vi "Program.vi"() -> ()   [LabVIEW 2023]
uses:
  <vilib>/measure/NI_MAPro.lvlib
  Controls/Enum 2 - States.ctl
  <vilib>/sound2/lvsound2.llb/Sampling Mode.ctl
  <vilib>/sound2/lvsound2.llb/Sound Input Task ID.ctl
  <vilib>/sound2/lvsound2.llb/Sound File Refnum.ctl
  Controls/Enum 1.ctl
  <vilib>/sound2/lvsound2.llb/Sound Data Format.ctl
  Controls/Enum 3 - States.ctl
  Controls/UI Message.ctl
  <vilib>/sound2/lvsound2.llb/Sound Input Read (DBL).vi
  <vilib>/measure/maspectr.llb/FFT Spectrum (Mag-Phase) for N Chan.vi
  <vilib>/sound2/lvsound2.llb/Sound File Write Open.vi
  <vilib>/sound2/lvsound2.llb/Sound File Write (DBL).vi
  Controls/Parameters In.ctl
panel:
  in  "Stop":bool
  in  "Sound format":T1={"sample rate (S/s)"=48000.0, "number of channels"=2, "bits per sample"=24}
  in  "number of samples/ch":i32=12000
  in  "Play":bool
  in  "Path":path
  in  "Tab Control":enum32{"Waveform Analyzer", "Spectrum Analyzer"}(tab)
  out "Waveform Graph":waveform(dbl)[](graph)
  out "Spectrum Graph":cluster{"f0":dbl, "df":dbl, "magnitude":dbl[]}[](graph)
  in  "Zoom 2":i32(slide) scale=100.0..1.0
  in  "Zoom":i32(slide) scale=1000.0..1.0
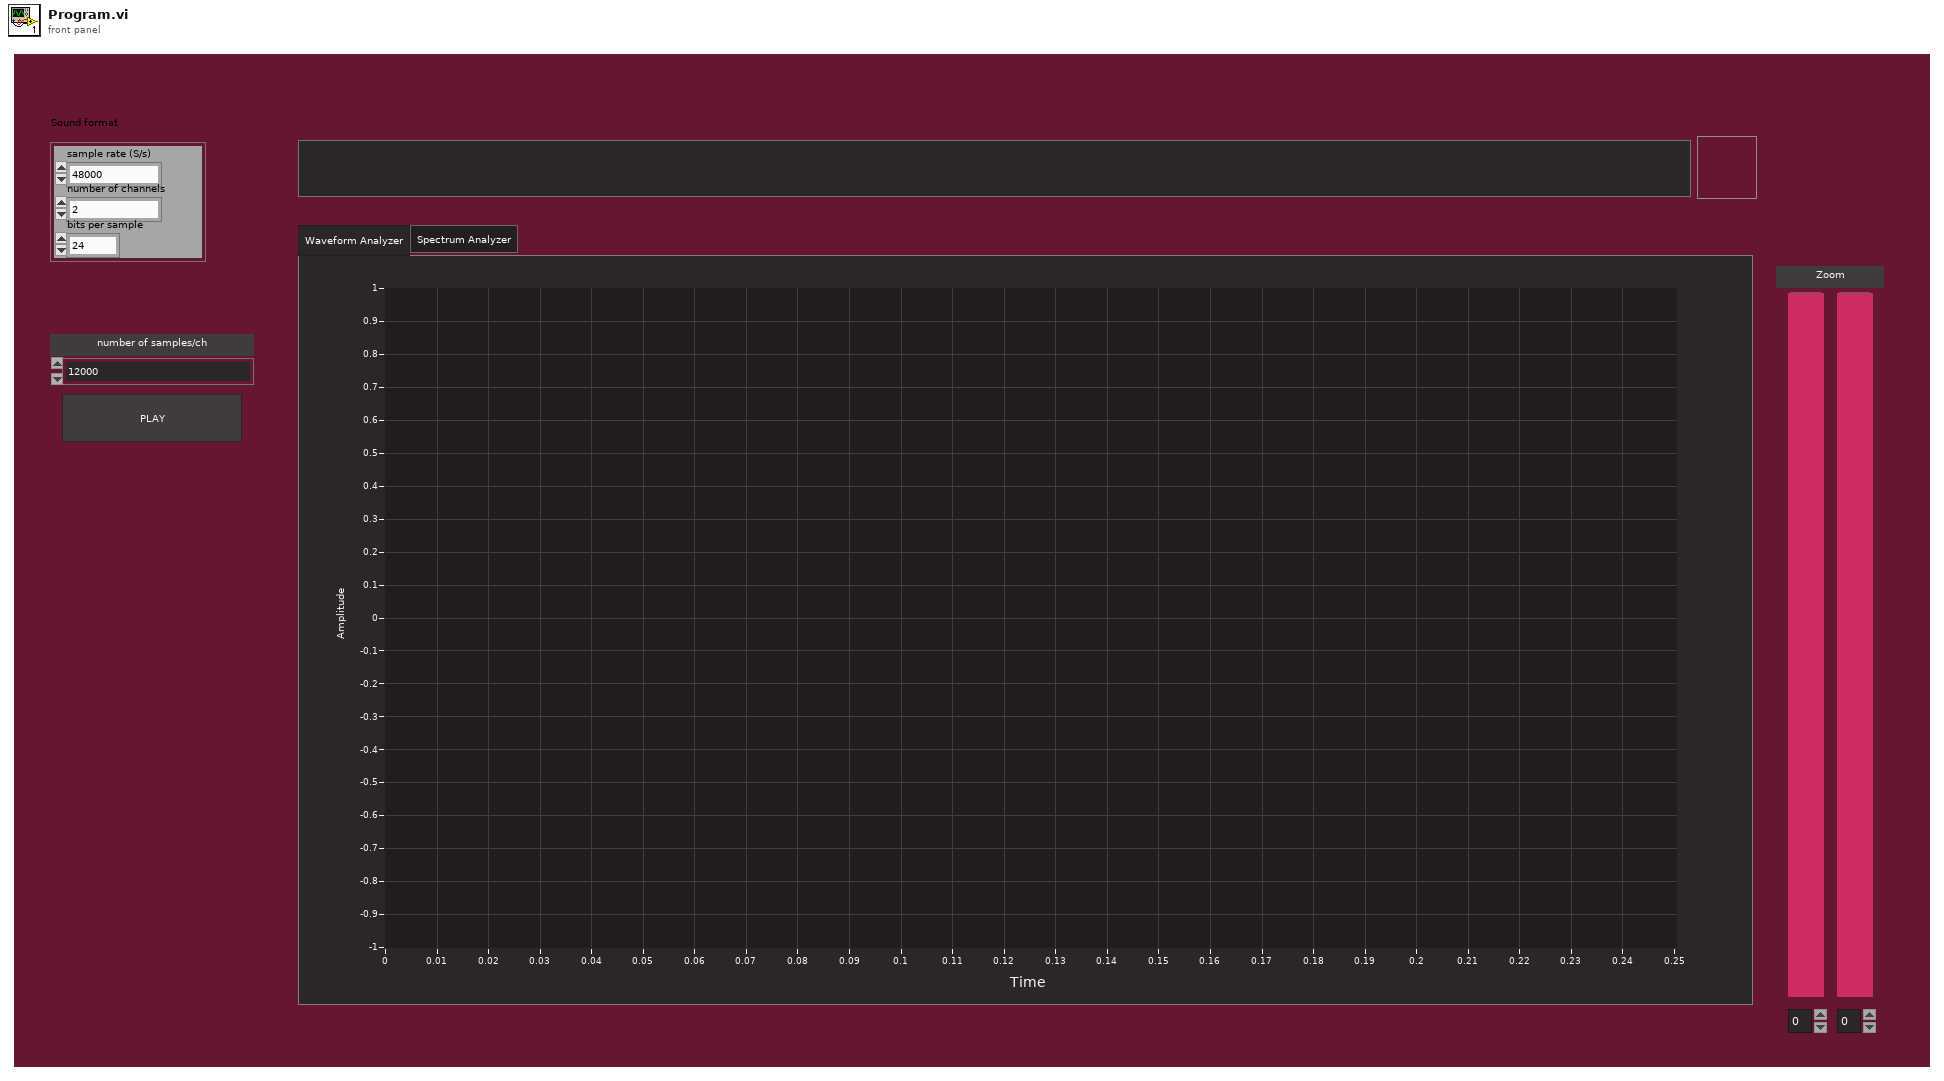
[diagram p1: front panel]
types:
  T1 = typedef "Sound Data Format.ctl" = cluster{"sample rate (S/s)":dbl, "number of channels":i32, "bits per sample":i32}
  T2 = typedef "UI Message.ctl" = cluster{"Time Signal ":waveform(dbl)[], "FFT":cluster{"f0":dbl, "df":dbl, "magnitude":dbl[]}[]}
  T3 = typedef "Enum 3 - States.ctl" = enum16{"Idle", "Init", "Analysis", "End"}
  T4 = typedef "Enum 2 - States.ctl" = enum16{"Idle", "Init", "ACQ", "End"}
  T5 = typedef "Parameters In.ctl" = cluster{"Stop":bool, "Play":bool, "number of samples/ch":i32, "sound format":T1, "Path":path}
  T6 = typedef "Enum 1.ctl" = enum16{"Set", "Get"}
  T7 = typedef "Sound File Refnum.ctl" = refnum<file>
  T8 = typedef "Sound Input Task ID.ctl" = u32
  T9 = typedef "Sampling Mode.ctl" = i32
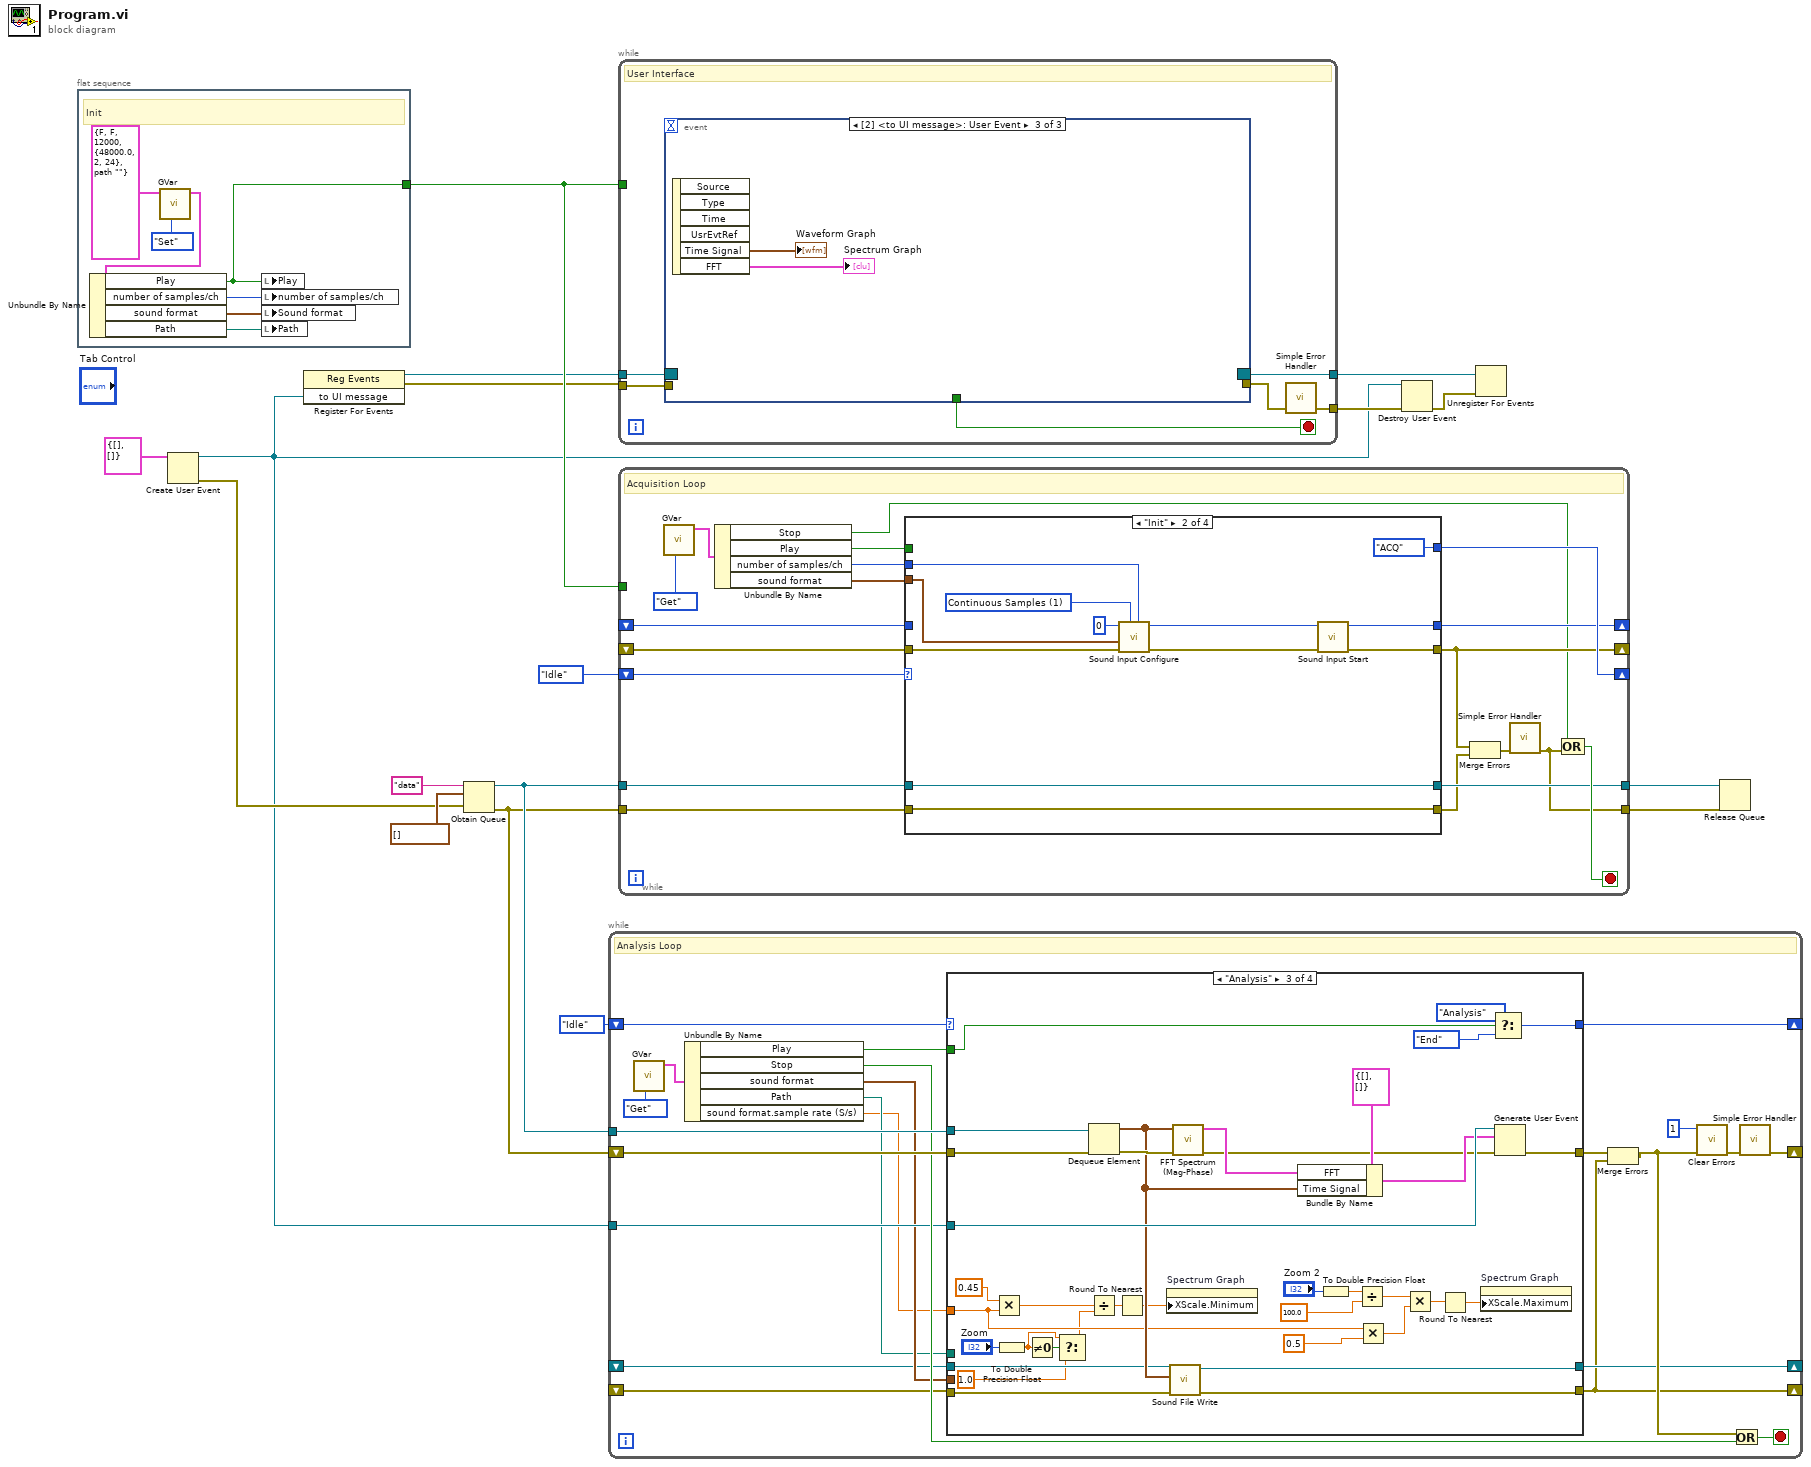
[diagram p0: block diagram]
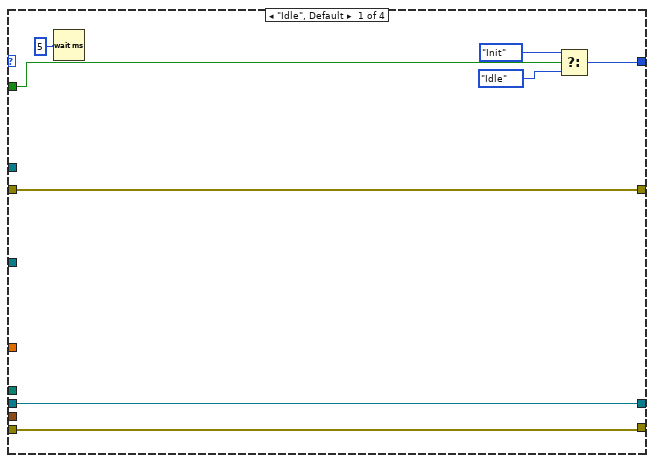
[diagram p2: hidden frame]
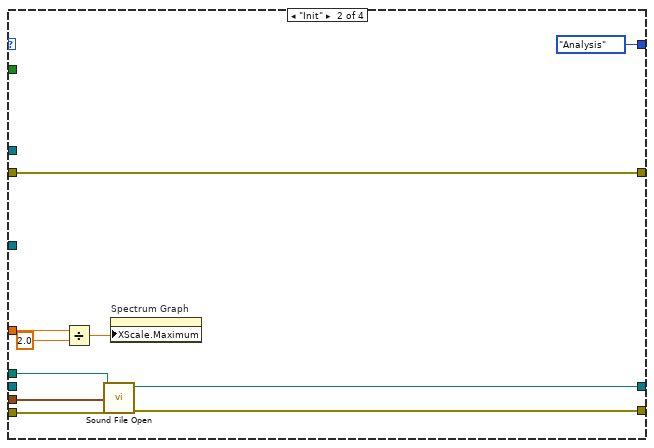
[diagram p3: hidden frame]
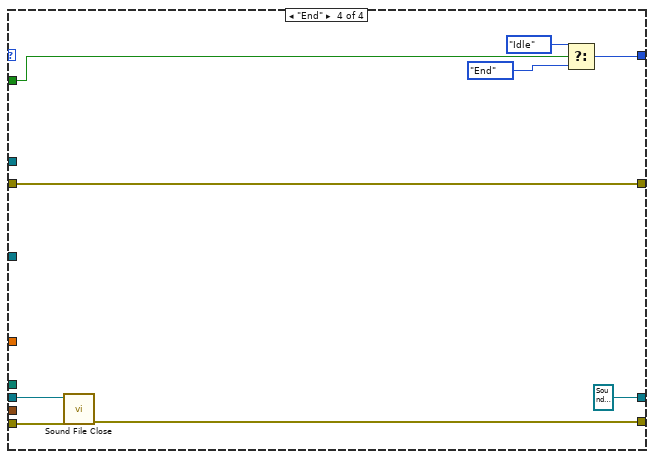
[diagram p4: hidden frame]
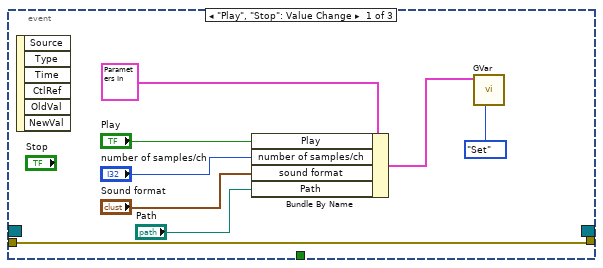
[diagram p5: hidden frame]
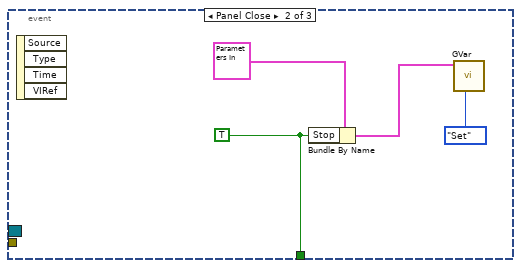
[diagram p6: hidden frame]
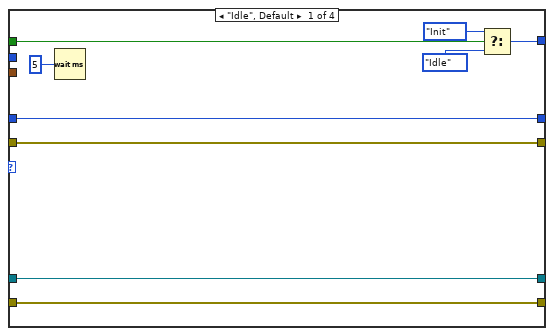
[diagram p7: hidden frame]
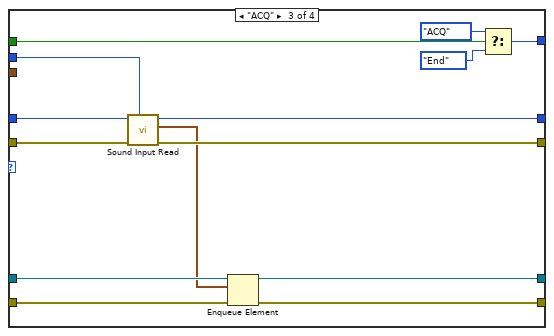
[diagram p8: hidden frame]
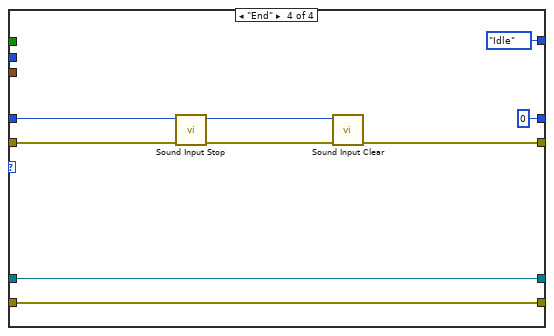
[diagram p9: hidden frame]
diagram:
  n1 = flat-sequence {
    tunnel: [w20] -> w16
    frame #0 {
      # "Init"
      n2 = call "GVar.vi"("Action"=Enum_1."Set", "Parameters In"=T5 {"Stop"=FALSE, "Play"=FALSE, "number of samples/ch"=12000, "sound format"={"sample rate (S/s)"=48000.0, "number of channels"=2, "bits per sample"=24}, "Path"=path ""}) -> ("Parameters In 2"=w23:T5)  [unwired: 9 in]
      n3 = Unbundle By Name(w23) -> ("Play"=w20:bool, "number of samples/ch"=w21:i32, "sound format"=w22:T1, "Path"=w19:path)
      n4 = local write "Play"(w20) -> ()
      n5 = local write "number of samples/ch"(w21) -> ()
      n6 = local write "Sound format"(w22) -> ()
      n7 = local write "Path"(w19) -> ()
    }
  }
  n8 = Create User Event(user event datatype=T2 {"Time Signal "=[], "FFT"=[]} ("to UI message")) -> (user event=w4:refnum<user-event>, error out=w11:errorcluster)  [unwired: 1 in]
  n9 = register-events(w4) -> (reference out=w10:refnum<event-registration>, error out=w7:errorcluster)  [unwired: 2 in]
  n10 = Obtain Queue(name (unnamed)="data", element data type=waveform(dbl)[] [] ("data"), error in (no error)=w11) -> (queue out=w13:refnum<queue>, error out=w1:errorcluster)  [unwired: 2 in, 1 out]
  n11 = while {
    tunnel: w13 -> [w45]
    shift-right: [w36] -> _
    shift-left: w1 -> [w44]
    shift-right: [w39] -> _
    shift-left: Enum_3_-_States."Idle" -> [w46]
    tunnel: w4 -> [w37]
    shift-right: [w31] -> _
    shift-left: _ -> [w27]
    shift-right: [w29] -> _
    shift-left: _ -> [w28]
    stop <- w41 stop-if-true
    # "Analysis Loop"
    n12 = call "GVar.vi"("Action"=Enum_1."Get") -> ("Parameters In 2"=w42:T5)  [unwired: 10 in]
    n13 = Unbundle By Name(w42) -> ("Play"=w38:bool, "Stop"=w40:bool, "sound format"=w33:T1, "Path"=w26:path, "sound format.sample rate (S/s)"=w25:dbl)
    n14 = case shown="\"Analysis\"" w46 {
      tunnel: w44 -> [w53 w62 w100 w101]
      tunnel: w45 -> [_ _ w99 _]
      tunnel: [w53 w62 w88 w101] -> w30
      tunnel: [w50 Enum_3_-_States."Analysis" w95 w107] -> w39
      tunnel: w38 -> [w49 _ w94 w106]
      tunnel: w37 -> [_ _ w93 _]
      tunnel: w33 -> [_ w64 _ _]
      tunnel: [w47 w63 w84 T7 refnum ("sound file refnum out")] -> w31
      tunnel: [w48 w61 w86 w103] -> w29
      tunnel: w28 -> [w48 w59 w83 w104]
      tunnel: w27 -> [w47 _ w85 w105]
      tunnel: w26 -> [_ w58 _ _]
      tunnel: w25 -> [_ w57 w70 _]
      frame "Idle", Default {
        n15 = Wait (ms)(milliseconds to wait=u32 5) -> ()  [unwired: 1 out]
        n16 = Select(t=Enum_3_-_States."Init", s=w49, f=Enum_3_-_States."Idle") -> (s? t:f=w50:T3)
      }
      frame "Init" {
        n17 = Divide(x=w57, y=2.0) -> (x/y=w55:dbl)
        n18 = call-poly <vilib>:"Sound File Open.vi"("error in (no error)"=w59, "sound format"=w64, "path"=w58) -> ("error out"=w61:errorcluster, "sound file refnum"=w63:T7)  [unwired: 7 in]
        n19 = property on="Spectrum Graph" class="WFGraph (strict)"("XScale.Maximum"=w55) -> ()  [unwired: 2 in, 2 out]
      }
      frame "Analysis" {
        n20 = Multiply(x=0.45, y=w70) -> (x*y=w81:dbl)
        n21 = To Double Precision Float(number="Zoom") -> (double precision float=w67:dbl)
        n22 = Not Equal To 0?(x=w67) -> (x != 0?=w68:bool)
        n23 = Select(t=w67, s=w68, f=1.0) -> (s? t:f=w65:dbl)
        n24 = Dequeue Element(queue=w99, error in (no error)=w100) -> (element=w87:waveform(dbl)[], error out=w98:errorcluster)  [unwired: 1 in, 2 out]
        n25 = Divide(x=w81, y=w65) -> (x/y=w73:dbl)
        n26 = Round To Nearest(number=w73) -> (nearest integer value=w72:dbl)
        n27 = property on="Spectrum Graph" class="WFGraph (strict)"("XScale.Minimum"=w72) -> ()  [unwired: 2 in, 2 out]
        n28 = call-poly <vilib>:"Sound File Write.vi"("error in (no error)"=w83, "data"=w87, "sound file refnum"=w85) -> ("error out"=w86:errorcluster, "sound file refnum out"=w84:T7)  [unwired: 7 in]
        n29 = call-poly <vilib>:"FFT Spectrum (Mag-Phase).vi"("error in (no error)"=w98, "time signals"=w87) -> ("error out"=w89:errorcluster, "magnitudes"=w92:cluster{"f0":dbl, "df":dbl, "magnitude":dbl[]}[])  [unwired: 5 in, 3 out]
        n30 = Bundle By Name(cluster=T2 {"Time Signal "=[], "FFT"=[]} ("to UI message"), "FFT"=w92, "Time Signal"=w87) -> (w90:T2)
        n31 = To Double Precision Float(number="Zoom 2") -> (double precision float=w77:dbl)
        n32 = Divide(x=w77, y=100.0) -> (x/y=w80:dbl)
        n33 = Multiply(x=w70, y=0.5) -> (x*y=w69:dbl)
        n34 = Multiply(x=w80, y=w69) -> (x*y=w75:dbl)
        n35 = Round To Nearest(number=w75) -> (nearest integer value=w74:dbl)
        n36 = property on="Spectrum Graph" class="WFGraph (strict)"("XScale.Maximum"=w74) -> ()  [unwired: 2 in, 2 out]
        n37 = Select(t=Enum_3_-_States."Analysis", s=w94, f=Enum_3_-_States."End") -> (s? t:f=w95:T3)
        n38 = Generate User Event(user event=w93, event data cluster=w90, error in=w89) -> (error out=w88:errorcluster)  [unwired: 1 in, 1 out]
      }
      frame "End" {
        n39 = call <vilib>:"Sound File Close.vi"("error in (no error)"=w104, "sound file refnum"=w105) -> ("error out"=w103:errorcluster)  [unwired: 9 in]
        n40 = Select(t=Enum_3_-_States."Idle", s=w106, f=Enum_3_-_States."End") -> (s? t:f=w107:T3)
      }
    }
    n41 = Merge Errors(w30, w29) -> (w32:errorcluster)
    n42 = call <vilib>:"Clear Errors.vi"("error in (no error)"=w32, "specific error code to clear (0: all)"=1) -> ("error out"=w34:errorcluster)  [unwired: 4 in, 1 out]
    n43 = Or(x=w32, y=w40) -> (x .or. y?=w41:bool)
    n44 = call <vilib>:"Simple Error Handler.vi"("error in (no error)"=w34) -> ("error out"=w36:errorcluster)  [unwired: 4 in, 4 out]
  }
  n45 = while {
    tunnel: w16 -> [_]
    tunnel: w10 -> [w114]
    tunnel: [w113] -> w8
    tunnel: w7 -> [w112]
    tunnel: [w110] -> w6
    stop <- w115 stop-if-true
    # "User Interface"
    n46 = event shown="[2] <to UI message>: User Event" {
      selector: w114 -> [_ _ _]
      dyn-events: [_ _ _] -> w113
      timeout: _ -> [_ _ _]
      tunnel: [_ w126 _] -> w115
      tunnel: [w122 _ _] -> w111
      tunnel: w112 -> [w122 _ _]
      event "Play", "Stop": Value Change {
        n47 = event-data() -> ()  [unwired: 1 in, 6 out]
        n48 = Bundle By Name(cluster=T5 {"Stop"=FALSE, "Play"=FALSE, "number of samples/ch"=12000, "sound format"={"sample rate (S/s)"=48000.0, "number of channels"=2, "bits per sample"=24}, "Path"=path ""} ("Parameters In"), "Play"="Play", "number of samples/ch"="number of samples/ch", "sound format"="Sound format", "Path"="Path") -> (w116:T5)
        n49 = call "GVar.vi"("Action"=Enum_1."Set", "Parameters In"=w116) -> ()  [unwired: 9 in, 1 out]
      }
      event Panel Close {
        w126 = TRUE
        n50 = event-data() -> ()  [unwired: 1 in, 4 out]
        n51 = Bundle By Name(cluster=T5 {"Stop"=FALSE, "Play"=FALSE, "number of samples/ch"=12000, "sound format"={"sample rate (S/s)"=48000.0, "number of channels"=2, "bits per sample"=24}, "Path"=path ""} ("Parameters In"), "Stop"=w126) -> (w124:T5)
        n52 = call "GVar.vi"("Action"=Enum_1."Set", "Parameters In"=w124) -> ()  [unwired: 9 in, 1 out]
      }
      event User Event {
        n53 = event-data() -> ("Time Signal"=→"Waveform Graph":waveform(dbl)[], "FFT"=→"Spectrum Graph":cluster{"f0":dbl, "df":dbl, "magnitude":dbl[]}[])  [unwired: 1 in, 4 out]
      }
    }
    n54 = call <vilib>:"Simple Error Handler.vi"("error in (no error)"=w111) -> ("error out"=w110:errorcluster)  [unwired: 4 in, 4 out]
  }
  n55 = while {
    shift-right: [w147] -> _
    shift-left: Enum_2_-_States."Idle" -> [w148]
    shift-right: [w146] -> _
    shift-left: _ -> [w144]
    shift-right: [w137] -> _
    shift-left: _ -> [w145]
    tunnel: w16 -> [_]
    tunnel: w13 -> [w140]
    tunnel: w1 -> [w139]
    tunnel: [w134] -> w2
    tunnel: [w138] -> w3
    stop <- w143 stop-if-true
    # "Acquisition Loop"
    n56 = call "GVar.vi"("Action"=Enum_1."Get") -> ("Parameters In 2"=w142:T5)  [unwired: 10 in]
    n57 = Unbundle By Name(w142) -> ("Stop"=w133:bool, "Play"=w132:bool, "number of samples/ch"=w130:i32, "sound format"=w131:T1)
    n58 = case shown="\"Init\"" w148 {
      tunnel: [w155 Enum_2_-_States."ACQ" ("f") w179 Enum_2_-_States."Idle"] -> w147
      tunnel: [w152 w166 w183 T8 0 ("task ID out")] -> w146
      tunnel: [w153 w163 w182 w186] -> w137
      tunnel: w145 -> [w153 w158 w175 w191]
      tunnel: w144 -> [w152 _ w176 w189]
      tunnel: w132 -> [w154 _ w181 _]
      tunnel: w130 -> [_ w162 w177 _]
      tunnel: w131 -> [_ w161 _ _]
      tunnel: w140 -> [w151 w160 w174 w184]
      tunnel: w139 -> [w150 w159 w173 w185]
      tunnel: [w150 w159 w172 w185] -> w135
      tunnel: [w151 w160 w171 w184] -> w138
      frame "Idle", Default {
        n59 = Wait (ms)(milliseconds to wait=u32 5) -> ()  [unwired: 1 out]
        n60 = Select(t=Enum_2_-_States."Init", s=w154, f=Enum_2_-_States."Idle") -> (s? t:f=w155:T4)
      }
      frame "Init" {
        w169 = T9 1 items=["Finite Samples", "Continuous Samples"] ("sample mode")
        n61 = call <vilib>:"Sound Input Configure.vi"("number of samples/ch"=w162, "sample mode"=w169, "error in (no error)"=w158, "sound format"=w161, "device ID"=u32 0) -> ("error out"=w165:errorcluster, "task ID"=w167:T8)  [unwired: 5 in]
        n62 = call <vilib>:"Sound Input Start.vi"("error in (no error)"=w165, "task ID"=w167) -> ("error out"=w163:errorcluster, "task ID out"=w166:T8)  [unwired: 8 in]
      }
      frame "ACQ" {
        n63 = call-poly <vilib>:"Sound Input Read.vi"("number of samples/ch"=w177, "error in (no error)"=w175, "task ID"=w176) -> ("error out"=w182:errorcluster, "data"=w170:waveform(dbl)[], "task ID out"=w183:T8)  [unwired: 6 in]
        n64 = Enqueue Element(queue=w174, element=w170, error in (no error)=w173) -> (queue out=w171:refnum<queue>, error out=w172:errorcluster)  [unwired: 1 in, 1 out]
        n65 = Select(t=Enum_2_-_States."ACQ", s=w181, f=Enum_2_-_States."End") -> (s? t:f=w179:T4)
      }
      frame "End" {
        n66 = call <vilib>:"Sound Input Stop.vi"("error in (no error)"=w191, "task ID"=w189) -> ("error out"=w188:errorcluster, "task ID out"=w192:T8)  [unwired: 8 in]
        n67 = call <vilib>:"Sound Input Clear.vi"("error in (no error)"=w188, "task ID"=w192) -> ("error out"=w186:errorcluster)  [unwired: 9 in]
      }
    }
    n68 = Merge Errors(w137, w135) -> (w136:errorcluster)
    n69 = call <vilib>:"Simple Error Handler.vi"("error in (no error)"=w136) -> ("error out"=w134:errorcluster)  [unwired: 4 in, 4 out]
    n70 = Compound Arithmetic op=OR(w133, w134) -> (w143:bool)
  }
  n71 = Destroy User Event(user event=w4, error in=w6) -> (error out=w5:errorcluster)
  n72 = Unregister For Events(event registration refnum=w8, error in=w5) -> ()  [unwired: 1 out]
  n73 = Release Queue(queue=w3, error in (no error)=w2) -> ()  [unwired: 1 in, 3 out]
